vi "QT_MatrixRotate.vi"(0 "In Matrix [3x3] (Identity)":dbl[][](array[numeric])=[[1.0, 0.0, 0.0], [0.0, 1.0, 0.0], [0.0, 0.0, 1.0]] format="%.2f", 7 "Angle [deg]":dbl format="%.2f", 11 "error in (no error)":errorcluster) -> (4 "Out Matrix":dbl[][](array[numeric])=[[1.0, 0.0, 0.0], [0.0, 1.0, 0.0], [0.0, 0.0, 1.0]] format="%.2f", 10 "Out Matrix as Vector":dbl[](array[numeric])=[1.0, 0.0, 0.0] format="%.2f", 15 "error out":errorcluster)   [LabVIEW 2024]
uses:
  <vilib>/Analysis/baseanly.llb/Real A x B.vi
  <vilib>/Analysis/NI_AALBase.lvlib
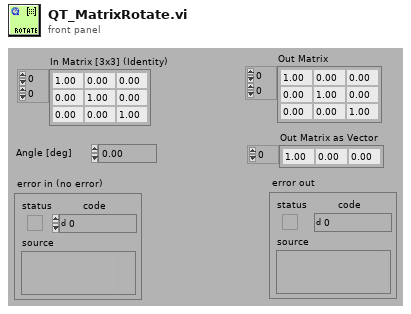
[diagram p1: front panel]
types:
  T1 = typedef "NI_Matrix.lvlib/RealMatrix.ctl" = dbl[][]
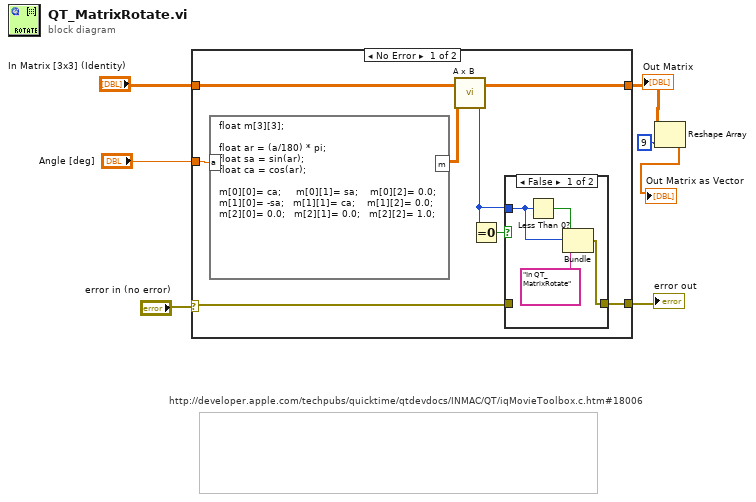
[diagram p0: block diagram]
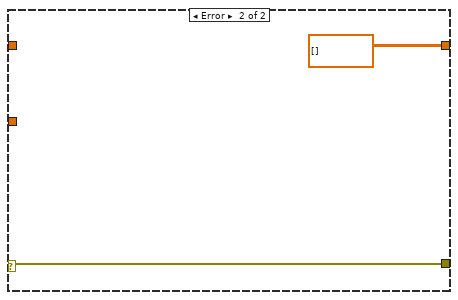
[diagram p3: hidden frame]
diagram:
  # "http://developer.apple.com/techpubs/quicktime/qtdevdocs/INMAC/QT/iqMovieToolbox.c.htm#18006"
  n1 = case shown="No Error" "error in (no error)" {
    selector: "error in (no error)" -> [w8 w21]
    tunnel: [w15 dbl[][] [] ("A x B")] -> w7
    tunnel: "In Matrix [3x3] (Identity)" -> [w14 _]
    tunnel: "Angle [deg]" -> [w12 _]
    tunnel: [w11 w21] -> w3
    frame No Error {
      n2 = formula code="float m[3][3];\n\nfloat ar = (a/180) * pi;\nfloat sa = sin(ar);\nfloat ca = cos(ar);\n\nm[0][0]= ca;     m[0][1]= sa;    m[0][2]= 0.0;\nm[1][0]= -sa;   m[1][1]= ca;    m[1][2]= 0.0;\nm[2][0]= 0.0;   m[2][1]= 0.0;   m[2][2]= 1.0;"("a"=w12) -> ("m"=w13:dbl[][])
      n3 = call-poly <vilib>:"A x B.vi"("B"=w13, "A"=w14) -> ("error"=w10:i32, "A x B"=w15:T1)
      n4 = Equal To 0?(x=w10) -> (x = 0?=w9:bool)
      n5 = case shown="False" w9 {
        tunnel: [w19 w20] -> w11
        tunnel: w10 -> [w17 _]
        tunnel: w8 -> [_ w20]
        frame False {
          n6 = Less Than 0?(x=w17) -> (x < 0?=w18:bool)
          n7 = Bundle(w18, "error"=w17, "In QT_MatrixRotate") -> (w19:cluster{bool, "error":i32, string})  [unwired: 1 out]
        }
        frame True {
        }
      }
    }
    frame Error {
    }
  }
  "Out Matrix" <- w7
  "error out" <- w3
  n8 = Reshape Array(w7, 9 ("dimension size")) -> (→"Out Matrix as Vector":dbl[])
